vi "GetSetManualRamp.vi"(0 "VISA resource name":refnum<visa-resource-name>, 5 "get/set":T2=enum."set", 7 "Channel Number (1-4)":T1=1 items=["Channel 1"=1, "Channel 2"=2, "Channel 3"=3, "Channel 4"=4], 9 "Set manual ramp":sgl format="%0.3f", 11 "error in":errorcluster) -> (4 "VISA resource name out":refnum<visa-resource-name>, 6 "Manual ramp setting string":string, 8 "Get manual ramp setting":sgl, 15 "error out":errorcluster)   [LabVIEW 2023, in "Thermotron 8800.lvlib"]
doc: "MRMP\nCommand name: Send or load manual ramp setting\nCommand type: Variable\nDescription: This is a manual mode command. The query command reads the manual ramp setting for the selected channel in units per minute. The units are in the scale selected at the 8800 (such as °C, °F, torr, %RH, etc.).\nSyntax: MRMPn? or MRMPn,data\nWhere n is any control channel (1 through 4) and data is the manual ramp rate.\nData type: Integer\nQuery example: MRMP2?\n8800 response: 30 (The manual ramp for channel 2 is 30 units per minute.)\nOperation example: MRMP1,12\n8800 response: The 8800 sets the manual ramp for channel 1 to 12 units per minute."
uses:
  Thermotron 8800.lvlib
  Private/get set.ctl
  Private/AnalogInputChannelNumber 1-4.ctl
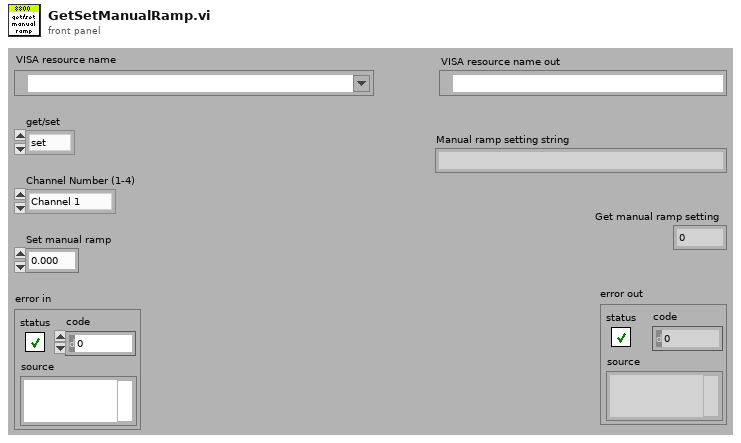
[diagram p1: front panel]
types:
  T1 = typedef "Thermotron 8800.lvlib/AnalogInputChannelNumber 1-4.ctl" = u16
  T2 = typedef "Thermotron 8800.lvlib/get set.ctl" = enum16{"get", "set"}
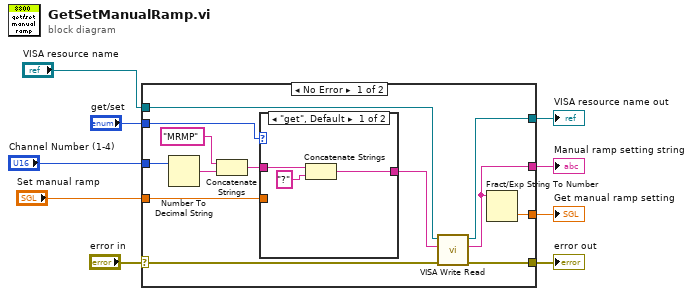
[diagram p0: block diagram]
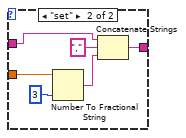
[diagram p2: hidden frame]
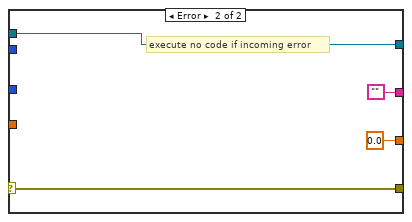
[diagram p3: hidden frame]
diagram:
  n1 = case shown="No Error" "error in" {
    selector: "error in" -> [w13 w35]
    tunnel: [w21 w35] -> w9
    tunnel: [w20 w34] -> w8
    tunnel: "VISA resource name" -> [w19 w34]
    tunnel: "Channel Number (1-4)" -> [w17 _]
    tunnel: "get/set" -> [w14 _]
    tunnel: [w11 ""] -> w4
    tunnel: "Set manual ramp" -> [w12 _]
    tunnel: [w10 0.0] -> w1
    frame No Error {
      n2 = Number To Decimal String(number=w17) -> (decimal integer string=w16:string)  [unwired: 1 in]
      n3 = Concatenate Strings("MRMP" ("8800 Command"), w16) -> (w15:string)
      n4 = case shown="\"get\", Default" w14 {
        tunnel: w15 -> [w24 w31]
        tunnel: [w25 w29] -> w22
        tunnel: w12 -> [_ w28]
        frame "get", Default {
          n5 = Concatenate Strings(w24, "?" ("8800 Command")) -> (w25:string)
        }
        frame "set" {
          n6 = Number To Fractional String(number=w28, precision (6)=i16 3) -> (F-format string=w27:string)  [unwired: 2 in]
          n7 = Concatenate Strings(w31, "," ("string"), w27) -> (w29:string)
        }
      }
      n8 = call "VISA Write Read.vi"("error in (no error)"=w13, "8800 Command"=w22, "VISA Refnum in"=w19) -> ("error out"=w21:errorcluster, "read buffer"=w11:string, "VISA Refnum out"=w20:refnum<visa-resource-name>)  [unwired: 6 in]
      n9 = Fract/Exp String To Number(string=w11) -> (number=w10:dbl)  [unwired: 3 in, 1 out]
    }
    frame Error {
      # "execute no code if incoming error"
    }
  }
  "VISA resource name out" <- w8
  "error out" <- w9
  "Manual ramp setting string" <- w4
  "Get manual ramp setting" <- w1
